vi "New.vi"   [LabVIEW 2024, in "Logging.lvlib" / "Data Item.lvclass"]
uses:
  Data Item.lvclass
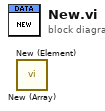
[diagram p0: block diagram]
diagram:
  n1 = call "New (Array).vi"() -> ()  [unwired: 10 in, 2 out]
  n2 = call "New (Element).vi"() -> ()  [unwired: 10 in, 2 out]
